vi "Initialize.vi"(8 "error in (no error)":errorcluster, 10 "Parameters in":refnum<class "Abstract Init Parameters.lvclass">, 11 "SLSC Switch Consumer in":refnum<class "SLSC Switch Consumer.lvclass">) -> (0 "error out":errorcluster, 3 "SLSC Switch Consumer out":refnum<class "SLSC Switch Consumer.lvclass">)   [LabVIEW 2016]
uses:
  Abstract Switch Init Parameters/Abstract Switch Init Parameters.lvclass
  SLSC Switch Consumer.lvclass
  Abstract Init Parameters/Abstract Init Parameters.lvclass
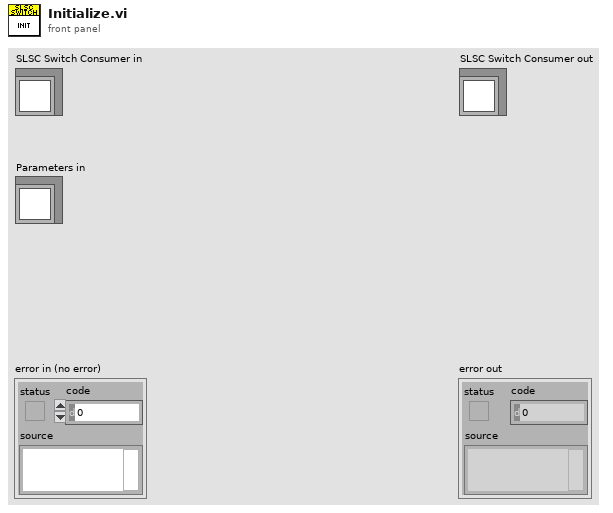
[diagram p1: front panel]
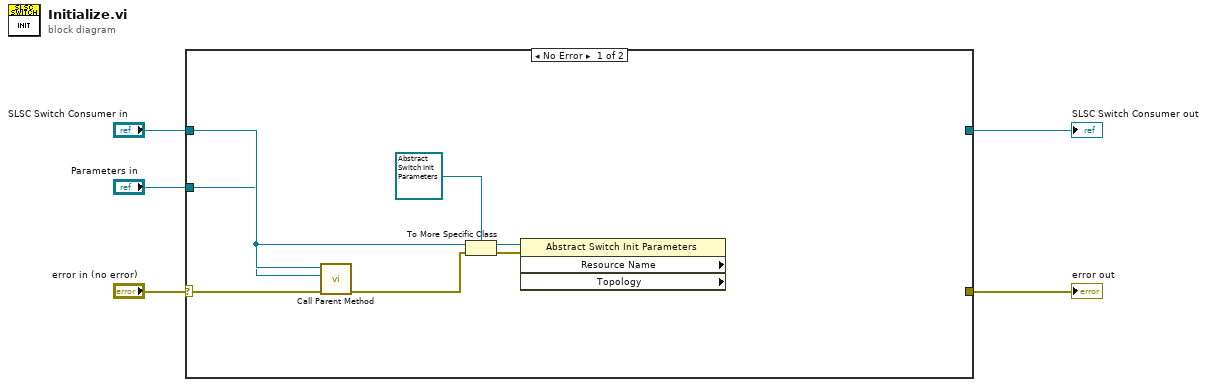
[diagram p0: block diagram]
diagram:
  n1 = case shown="No Error" "error in (no error)" {
    selector: "error in (no error)" -> [w14 w16]
    tunnel: [_ w16] -> w4
    tunnel: "SLSC Switch Consumer in" -> [w13 w15]
    tunnel: [w6 w15] -> w2
    tunnel: "Parameters in" -> [w10 _]
    frame No Error {
      n2 = call-parent "Call Parent Method"("error in (no error)"=w14, "Parameters in"=w10, "Abstract Switch Consumer in"=w13) -> ("error out"=w11:errorcluster, "Abstract Switch Consumer out"=w7:refnum<class "SLSC Switch Consumer.lvclass">)  [unwired: 7 in]
      n3 = To More Specific Class(target class=refnum<class "Abstract Switch Init Parameters.lvclass"> refnum ("Message Queue Library.lvlib:Abstract Switch Init Parameters.lvclass"), reference=w10, error in=w11) -> (specific class reference=w9:refnum<class "Abstract Switch Init Parameters.lvclass">, error out=w8:errorcluster)
      n4 = property class="Abstract Switch Init Parameters" props=["Resource Name", "Topology"](reference=w9, error in=w8) -> ()  [unwired: 4 out]
    }
    frame Error {
    }
  }
  "error out" <- w4
  "SLSC Switch Consumer out" <- w2
